vi "Run.vi"(8 "error in (no error)":errorcluster, 11 "Channel Req in":refnum<class "Channel Req.lvclass">) -> (0 "error out":errorcluster, 3 "Channel Req out":refnum<class "Channel Req.lvclass">)   [LabVIEW 2018, in "Channel Req.lvclass"]
uses:
  Channel Req.lvclass
  Socket/Socket.lvclass
  RxTx/RxTx.lvclass
  State Machine/State Machine.lvclass
  Communication Channel/Communication Channel.lvclass
  C:/Users/orlando/Documents/Orlando/communication-manager/communication-manager/Communication Channel/Communication Channel.lvclass
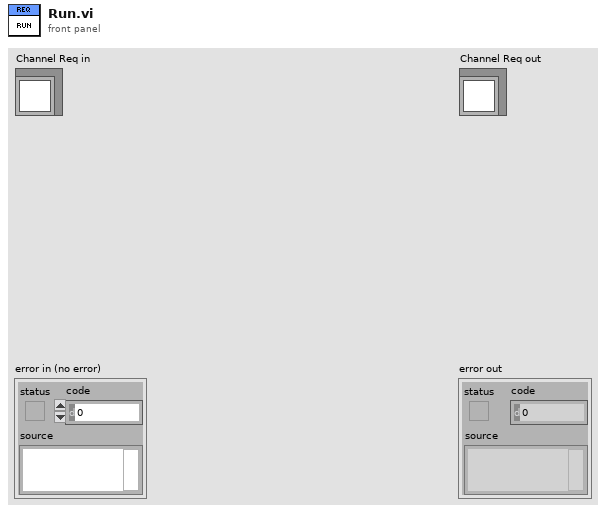
[diagram p1: front panel]
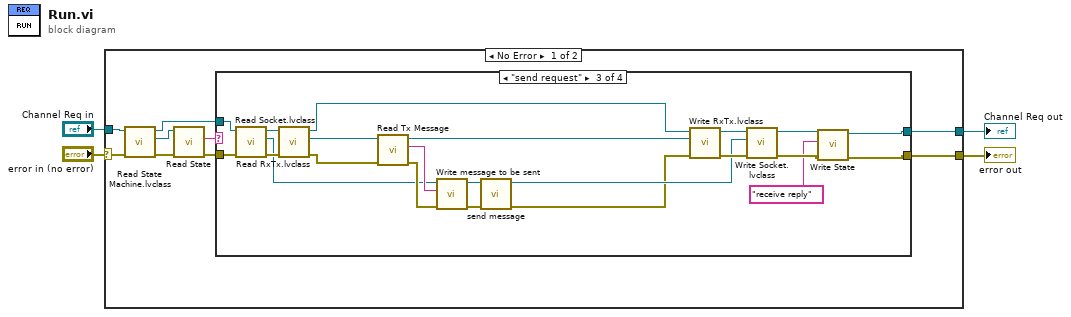
[diagram p0: block diagram]
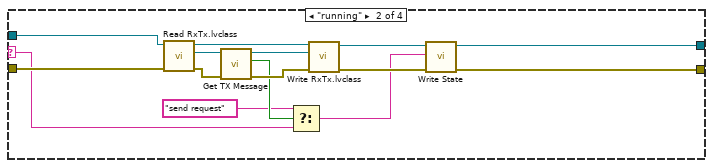
[diagram p3: hidden frame]
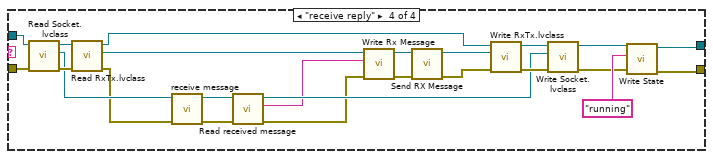
[diagram p4: hidden frame]
diagram:
  n1 = case shown="No Error" "error in (no error)" {
    selector: "error in (no error)" -> [w12 w77]
    tunnel: "Channel Req in" -> [w13 w78]
    tunnel: [w6 w78] -> w2
    tunnel: [w7 w77] -> w1
    frame No Error {
      n2 = call-dynamic "Read State Machine.lvclass.vi"("error in (no error)"=w12, "Communication Channel in"=w13) -> ("error out"=w11:errorcluster, "State Machine.lvclass"=w8:refnum<class "State Machine.lvclass">, "Communication Channel out"=w9:refnum<class "Channel Req.lvclass">)  [unwired: 7 in]
      n3 = call-dynamic "Read State.vi"("error in (no error)"=w11, "State Machine in"=w8) -> ("error out"=w5:errorcluster, "State"=w10:string)  [unwired: 7 in, 1 out]
      n4 = case shown="\"send request\"" w10 {
        selector: w10 -> [_ w18 _ _]
        tunnel: w9 -> [w15 w27 w52 w76]
        tunnel: [w15 w20 w34 w56] -> w6
        tunnel: [w14 w21 w32 w54] -> w7
        tunnel: w5 -> [w14 w26 w47 w71]
        frame Default {
        }
        frame "running" {
          n5 = call-dynamic "Read RxTx.lvclass.vi"("error in (no error)"=w26, "Communication Channel in"=w27) -> ("error out"=w28:errorcluster, "RxTx.lvclass"=w29:refnum<class "RxTx.lvclass">, "Communication Channel out"=w30:refnum<class "Channel Req.lvclass">)  [unwired: 7 in]
          n6 = call "Get TX Message.vi"("error in (no error)"=w28, "RxTx in"=w29) -> ("error out"=w24:errorcluster, "New msg"=w19:bool, "RxTx out"=w25:refnum<class "RxTx.lvclass">)  [unwired: 7 in]
          n7 = Select(t="send request", s=w19, f=w18) -> (s? t:f=w16:string)
          n8 = call-dynamic "Write RxTx.lvclass.vi"("error in (no error)"=w24, "RxTx.lvclass"=w25, "Communication Channel in"=w30) -> ("error out"=w22:errorcluster, "Communication Channel out"=w23:refnum<class "Channel Req.lvclass">)  [unwired: 7 in]
          n9 = call "Write State.vi"("error in (no error)"=w22, "new state"=w16, "Communication Channel in"=w23) -> ("error out"=w21:errorcluster, "Communication Channel out"=w20:refnum<class "Communication Channel.lvclass">)  [unwired: 7 in]
        }
        frame "send request" {
          n10 = call-dynamic "Read Socket.lvclass.vi"("error in (no error)"=w47, "Communication Channel in"=w52) -> ("error out"=w50:errorcluster, "Socket.lvclass"=w41:refnum<class "Socket.lvclass">, "Communication Channel out"=w51:refnum<class "Channel Req.lvclass">)  [unwired: 7 in]
          n11 = call-dynamic "Read RxTx.lvclass.vi"("error in (no error)"=w50, "Communication Channel in"=w51) -> ("error out"=w39:errorcluster, "RxTx.lvclass"=w40:refnum<class "RxTx.lvclass">, "Communication Channel out"=w46:refnum<class "Channel Req.lvclass">)  [unwired: 7 in]
          n12 = call "Read Tx Message.vi"("error in (no error)"=w39, "RxTx in"=w40) -> ("error out"=w42:errorcluster, "Tx Message"=w43:string, "RxTx out"=w36:refnum<class "RxTx.lvclass">)  [unwired: 7 in]
          n13 = call-dynamic "Write message to be sent.vi"("error in (no error)"=w42, "message to be sent"=w43, "Socket in"=w41) -> ("error out"=w44:errorcluster, "Socket out"=w45:refnum<class "Socket.lvclass">)  [unwired: 7 in]
          n14 = call "send message.vi"("error in (no error)"=w44, "Socket in"=w45) -> ("error out"=w37:errorcluster, "Socket out"=w38:refnum<class "Socket.lvclass">)  [unwired: 8 in]
          n15 = call-dynamic "Write RxTx.lvclass.vi"("error in (no error)"=w37, "RxTx.lvclass"=w36, "Communication Channel in"=w46) -> ("error out"=w48:errorcluster, "Communication Channel out"=w49:refnum<class "Channel Req.lvclass">)  [unwired: 7 in]
          n16 = call-dynamic "Write Socket.lvclass.vi"("error in (no error)"=w48, "Socket2.lvclass"=w38, "Communication Channel in"=w49) -> ("error out"=w33:errorcluster, "Communication Channel out"=w35:refnum<class "Channel Req.lvclass">)  [unwired: 7 in]
          n17 = call "Write State.vi"("error in (no error)"=w33, "new state"="receive reply", "Communication Channel in"=w35) -> ("error out"=w32:errorcluster, "Communication Channel out"=w34:refnum<class "Communication Channel.lvclass">)  [unwired: 7 in]
        }
        frame "receive reply" {
          n18 = call-dynamic "Read Socket.lvclass.vi"("error in (no error)"=w71, "Communication Channel in"=w76) -> ("error out"=w74:errorcluster, "Socket.lvclass"=w59:refnum<class "Socket.lvclass">, "Communication Channel out"=w75:refnum<class "Channel Req.lvclass">)  [unwired: 7 in]
          n19 = call-dynamic "Read RxTx.lvclass.vi"("error in (no error)"=w74, "Communication Channel in"=w75) -> ("error out"=w58:errorcluster, "RxTx.lvclass"=w60:refnum<class "RxTx.lvclass">, "Communication Channel out"=w70:refnum<class "Channel Req.lvclass">)  [unwired: 7 in]
          n20 = call-dynamic "receive message.vi"("error in (no error)"=w58, "Socket in"=w59) -> ("error out"=w68:errorcluster, "Socket out"=w69:refnum<class "Socket.lvclass">)  [unwired: 8 in]
          n21 = call-dynamic "Read received message.vi"("error in (no error)"=w68, "Socket in"=w69) -> ("error out"=w64:errorcluster, "received message"=w63:string, "Socket out"=w65:refnum<class "Socket.lvclass">)  [unwired: 7 in]
          n22 = call "Write Rx Message.vi"("error in (no error)"=w64, "Rx Message"=w63, "RxTx in"=w60) -> ("error out"=w61:errorcluster, "RxTx out"=w62:refnum<class "RxTx.lvclass">)  [unwired: 7 in]
          n23 = call "Send RX Message.vi"("error in (no error)"=w61, "RxTx in"=w62) -> ("error out"=w66:errorcluster, "RxTx out"=w67:refnum<class "RxTx.lvclass">)  [unwired: 8 in]
          n24 = call-dynamic "Write RxTx.lvclass.vi"("error in (no error)"=w66, "RxTx.lvclass"=w67, "Communication Channel in"=w70) -> ("error out"=w72:errorcluster, "Communication Channel out"=w73:refnum<class "Channel Req.lvclass">)  [unwired: 7 in]
          n25 = call-dynamic "Write Socket.lvclass.vi"("error in (no error)"=w72, "Socket2.lvclass"=w65, "Communication Channel in"=w73) -> ("error out"=w55:errorcluster, "Communication Channel out"=w53:refnum<class "Channel Req.lvclass">)  [unwired: 7 in]
          n26 = call "Write State.vi"("error in (no error)"=w55, "new state"="running", "Communication Channel in"=w53) -> ("error out"=w54:errorcluster, "Communication Channel out"=w56:refnum<class "Communication Channel.lvclass">)  [unwired: 7 in]
        }
      }
    }
    frame Error {
    }
  }
  "error out" <- w1
  "Channel Req out" <- w2
